vi "QDMH POLY Enqueue Strings.vi"(8 "error in (no error)":errorcluster, 10 "States":string[](array[string]), 11 "queue":refnum<queue>) -> (0 "error out":errorcluster, 3 "queue out":refnum<queue>)   [LabVIEW 2011]
doc: "This is an instance VI for the polymorphic enqueue VI.\n\nAAL 9/09"
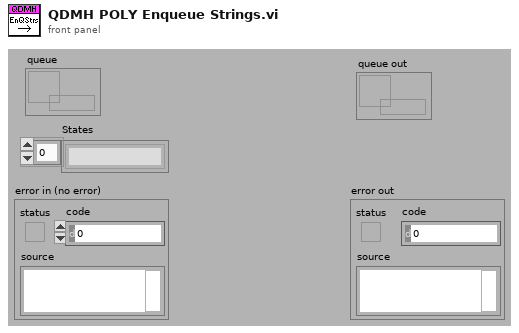
[diagram p1: front panel]
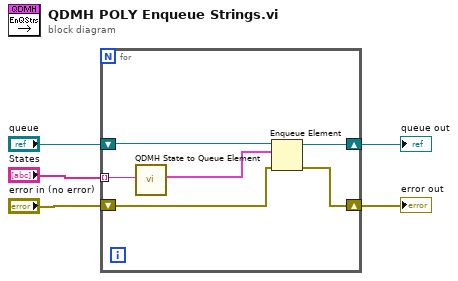
[diagram p0: block diagram]
diagram:
  n1 = for {
    tunnel: "States" -> [w6] mode=indexing
    shift-right: [w10] -> w4
    shift-left: "queue" -> [w11]
    shift-right: [w7] -> w2
    shift-left: "error in (no error)" -> [w8]
    n2 = call "QDMH State to Queue Element.vi"("State"=w6) -> ("QDSM Element"=w9:cluster{"State":string, "Variant Data":variant})  [unwired: 10 out]
    n3 = Enqueue Element(queue=w11, element=w9, error in (no error)=w8) -> (queue out=w10:refnum<queue>, error out=w7:errorcluster)  [unwired: 2 out]
  }
  "queue out" <- w4
  "error out" <- w2
